vi "Shutdown.vi"() -> ()   [LabVIEW 2024, in "Application.lvlib"]
uses:
  Application.lvlib
  Support/General Type Defs/Global Data.vi
  Support/User Events/User Events - Destroy.vi
  Support/General Type Defs/General Type Definitions.lvlib
  Support/User Events/User Events.lvlib
panel:
  out "Execution:State":T1(ring)
  out "error out":errorcluster
  in  "error in":errorcluster
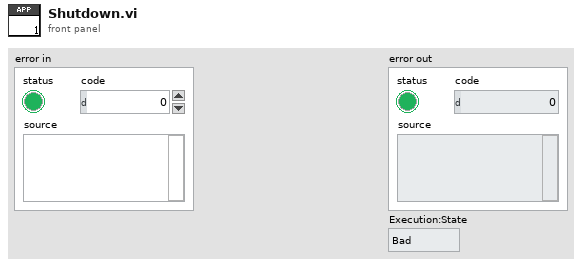
[diagram p1: front panel]
types:
  T1 = enum32{"Bad", "Idle", "Run top level", "Running"}
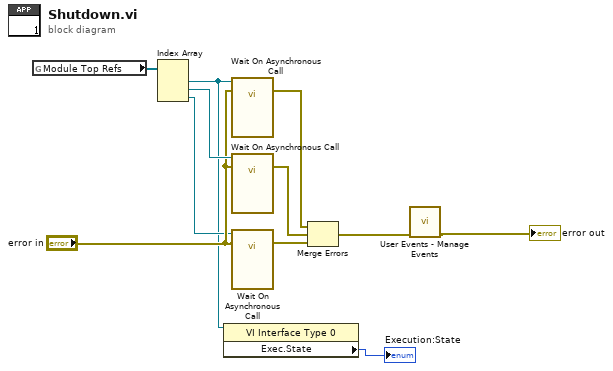
[diagram p0: block diagram]
diagram:
  n1 = global read "Global Data.vi" "Module Top Refs"() -> (w11:refnum<vi>[])
  n2 = Index Array(array=w11) -> (element #1=w1:refnum<vi>, element #2=w10:refnum<vi>, element #3=w3:refnum<vi>)  [unwired: 3 in]
  n3 = property class="VI Interface Type 0"(reference=w1) -> ("Exec.State"=→"Execution:State":T1)  [unwired: 1 in, 2 out]
  n4 = call-by-ref "Wait On Asynchronous Call"(reference=w1, error in="error in") -> (error out=w8:errorcluster)  [unwired: 11 in, 2 out]
  n5 = call-by-ref "Wait On Asynchronous Call"(reference=w10, error in="error in") -> (error out=w7:errorcluster)  [unwired: 11 in, 2 out]
  n6 = call-by-ref "Wait On Asynchronous Call"(reference=w3, error in="error in") -> (error out=w6:errorcluster)  [unwired: 11 in, 2 out]
  n7 = Merge Errors(w8, w7, w6) -> (w5:errorcluster)
  n8 = call-poly "User Events - Manage Events.vi"("error in"=w5) -> ("error out"=→"error out":errorcluster)  [unwired: 10 in]
